vi "Boolean - Error Message Contains String.vi"() -> ()   [LabVIEW 2017, in "Assertions.Tests.lvlib" / "Assert Is Not Boolean.lvlib"]
uses:
  Assert Is Not Boolean.lvlib
  src/Transparent Assertions/Assertions/Assertions.lvlib
panel:
  out "error out":errorcluster
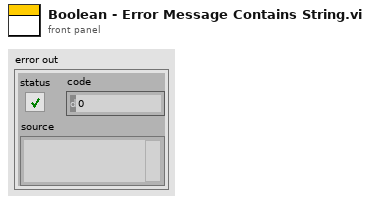
[diagram p1: front panel]
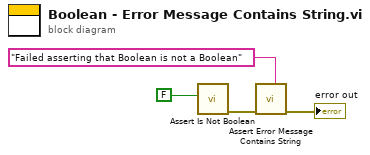
[diagram p0: block diagram]
diagram:
  n1 = call "Assert Is Not Boolean.vi"("Actual"=FALSE) -> ("error out"=w3:errorcluster)  [unwired: 10 in]
  n2 = call "Assert Error Message Contains String.vi"("Expected"="Failed asserting that Boolean is not a Boolean", "error in (no error)"=w3) -> ("error out"=→"error out":errorcluster)  [unwired: 9 in]
